vi "Create.vi"() -> (8 "File":refnum<class "File.lvclass">)   [LabVIEW 2020, in "File.lvclass"]
uses:
  File.lvclass
  File.lvclass/File.ctl
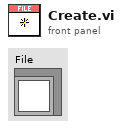
[diagram p1: front panel]
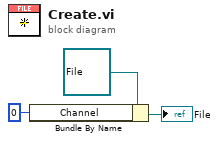
[diagram p0: block diagram]
diagram:
  n1 = Bundle By Name(cluster=refnum<class "File.lvclass"> refnum ("File"), "Channel"=0 ("Serialized.Channel")) -> (→"File":refnum<class "File.lvclass">)
